vi "Wrap_TPCANHandle.vi"(9 "Wram num to enum":bool, 10 "TPCANHandle numeric":u16 format="%x", 11 "TPCANHandle":T1) -> (2 "TPCANHandle out":T1, 3 "TPCANHandle out numeric":u16 format="%x")   [LabVIEW 2016]
doc: "Wrap TPCANHandle ENUM to numeric and vice versa."
uses:
  <instrlib>/KDI Digital Instrumentation/API_for_PCAN_BASIC_FD/TPCANHandle.ctl
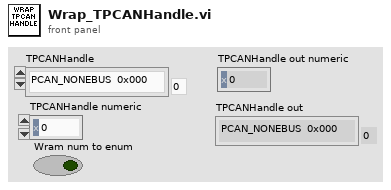
[diagram p1: front panel]
types:
  T1 = typedef "TPCANHandle.ctl" = enum16{"PCAN_NONEBUS  0x000", "PCAN_ISABUS1  0x21", "PCAN_ISABUS2  0x22", "PCAN_ISABUS3  0x23", "PCAN_ISABUS4  0x24", "PCAN_ISABUS5  0x25", "PCAN_ISABUS6  0x26", "PCAN_ISABUS7  0x27", "PCAN_ISABUS8  0x28", "PCAN_DNGBUS1  0x31", "PCAN_PCIBUS1  0x41", "PCAN_PCIBUS1  0x42", "PCAN_PCIBUS1  0x43", "PCAN_PCIBUS1  0x44", "PCAN_PCIBUS1  0x45", "PCAN_PCIBUS1  0x46", "PCAN_PCIBUS1  0x47", "PCAN_PCIBUS1  0x48", "PCAN_PCIBUS1  0x409", "PCAN_PCIBUS1  0x40A", "PCAN_PCIBUS1  0x40B", "PCAN_PCIBUS1  0x40C", "PCAN_PCIBUS1  0x40D", "PCAN_PCIBUS1  0x40E", "PCAN_PCIBUS1  0x40F", "PCAN_PCIBUS1  0x410", "PCAN_USBBUS1  0x51", "PCAN_USBBUS2  0x52", "PCAN_USBBUS3  0x53", "PCAN_USBBUS4  0x54", "PCAN_USBBUS5  0x55", "PCAN_USBBUS6  0x56", "PCAN_USBBUS7  0x57", "PCAN_USBBUS8  0x58", "PCAN_USBBUS9  0x509", "PCAN_USBBUS10  0x50A", "PCAN_USBBUS11  0x50B", "PCAN_USBBUS12  0x50C", "PCAN_USBBUS13  0x50D", "PCAN_USBBUS14  0x50E", "PCAN_USBBUS15  0x50F", "PCAN_USBBUS16  0x510", "PCAN_PCCBUS1  0x61", "PCAN_PCCBUS2  0x62", "PCAN_LANBUS1  0x801", "PCAN_LANBUS2  0x802", "PCAN_LANBUS3  0x803", "PCAN_LANBUS4  0x804", "PCAN_LANBUS5  0x805", "PCAN_LANBUS6  0x806", "PCAN_LANBUS7  0x807", "PCAN_LANBUS8  0x808", "PCAN_LANBUS9  0x809", "PCAN_LANBUS10  0x80A", "PCAN_LANBUS11  0x80B", "PCAN_LANBUS12  0x80C", "PCAN_LANBUS13  0x80D", "PCAN_LANBUS14  0x80E", "PCAN_LANBUS15  0x80F", "PCAN_LANBUS16  0x810"}
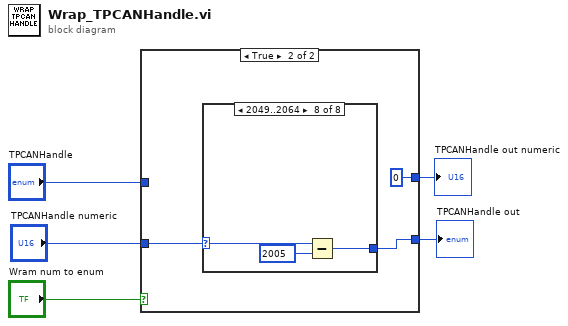
[diagram p0: block diagram]
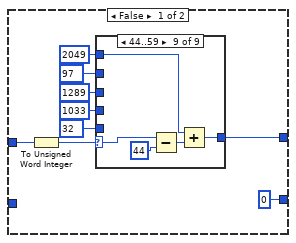
[diagram p2: hidden frame]
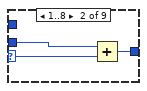
[diagram p4: hidden frame]
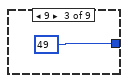
[diagram p5: hidden frame]
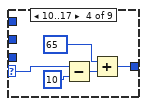
[diagram p6: hidden frame]
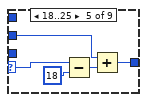
[diagram p7: hidden frame]
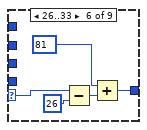
[diagram p8: hidden frame]
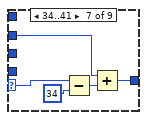
[diagram p9: hidden frame]
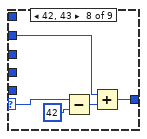
[diagram p10: hidden frame]
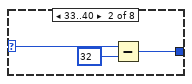
[diagram p12: hidden frame]
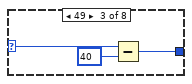
[diagram p13: hidden frame]
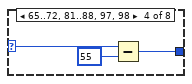
[diagram p14: hidden frame]
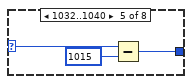
[diagram p15: hidden frame]
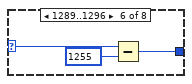
[diagram p16: hidden frame]
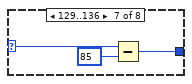
[diagram p17: hidden frame]
diagram:
  n1 = case shown="True" "Wram num to enum" {
    tunnel: [w8 u16 0] -> w5
    tunnel: "TPCANHandle" -> [w7 _]
    tunnel: [u16 0 ("TPCANHandle numeric") w50] -> w2
    tunnel: "TPCANHandle numeric" -> [_ w51]
    frame False {
      n2 = To Unsigned Word Integer(number=w7) -> (unsigned 16bit integer=w9:u16)
      n3 = case shown="44..59" w9 {
        selector: w9 -> [w15 w17 _ w23 w28 w33 w38 w43 w48]
        tunnel: [w15 w18 u16 49 w24 w29 w34 w39 w44 w49] -> w8
        tunnel: u16 32 -> [_ w16 _ _ _ _ _ _ _]
        tunnel: u16 1033 -> [_ _ _ _ w25 _ _ _ _]
        tunnel: u16 1289 -> [_ _ _ _ _ _ w35 _ _]
        tunnel: u16 97 -> [_ _ _ _ _ _ _ w40 _]
        tunnel: u16 2049 -> [_ _ _ _ _ _ _ _ w45]
        frame 0, Default {
        }
        frame 1..8 {
          n4 = Add(x=w16, y=w17) -> (x+y=w18:u16)
        }
        frame 9 {
        }
        frame 10..17 {
          n5 = Subtract(x=w23, y=u16 10) -> (x-y=w22:u16)
          n6 = Add(x=u16 65, y=w22) -> (x+y=w24:u16)
        }
        frame 18..25 {
          n7 = Subtract(x=w28, y=u16 18) -> (x-y=w27:u16)
          n8 = Add(x=w25, y=w27) -> (x+y=w29:u16)
        }
        frame 26..33 {
          n9 = Subtract(x=w33, y=u16 26) -> (x-y=w32:u16)
          n10 = Add(x=u16 81, y=w32) -> (x+y=w34:u16)
        }
        frame 34..41 {
          n11 = Subtract(x=w38, y=u16 34) -> (x-y=w37:u16)
          n12 = Add(x=w35, y=w37) -> (x+y=w39:u16)
        }
        frame 42, 43 {
          n13 = Subtract(x=w43, y=u16 42) -> (x-y=w42:u16)
          n14 = Add(x=w40, y=w42) -> (x+y=w44:u16)
        }
        frame 44..59 {
          n15 = Subtract(x=w48, y=u16 44) -> (x-y=w47:u16)
          n16 = Add(x=w45, y=w47) -> (x+y=w49:u16)
        }
      }
    }
    frame True {
      n17 = case shown="2049..2064" w51 {
        selector: w51 -> [w53 w56 w59 w62 w65 w68 w71 w74]
        tunnel: [w53 w54 w57 w60 w63 w66 w69 w72] -> w50
        frame 0, Default {
        }
        frame 33..40 {
          n18 = Subtract(x=w56, y=u16 32) -> (x-y=w54:u16)
        }
        frame 49 {
          n19 = Subtract(x=w59, y=u16 40) -> (x-y=w57:u16)
        }
        frame 65..72, 81..88, 97, 98 {
          n20 = Subtract(x=w62, y=u16 55) -> (x-y=w60:u16)
        }
        frame 1032..1040 {
          n21 = Subtract(x=w65, y=u16 1015) -> (x-y=w63:u16)
        }
        frame 1289..1296 {
          n22 = Subtract(x=w68, y=u16 1255) -> (x-y=w66:u16)
        }
        frame 129..136 {
          n23 = Subtract(x=w71, y=u16 85) -> (x-y=w69:u16)
        }
        frame 2049..2064 {
          n24 = Subtract(x=w74, y=u16 2005) -> (x-y=w72:u16)
        }
      }
    }
  }
  "TPCANHandle out numeric" <- w5
  "TPCANHandle out" <- w2
